vi "P1, P2, O2 Calculations.vi"(9 "O2 Voltage":dbl, 10 "P2 Voltage":dbl, 11 "P1 Voltage":dbl) -> (1 "O2":dbl, 2 "P2 Pressure":dbl, 3 "P1 Pressure":dbl)   [LabVIEW 2018]
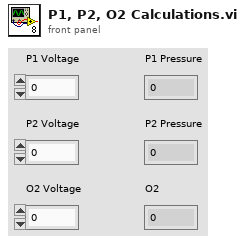
[diagram p1: front panel]
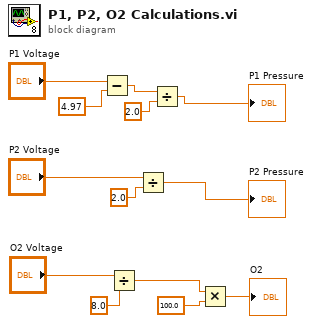
[diagram p0: block diagram]
diagram:
  n1 = Subtract(x="P1 Voltage", y=4.97 ("minimum value")) -> (x-y=w6:dbl)
  n2 = Divide(x="O2 Voltage", y=8.0 ("minimum value")) -> (x/y=w10:dbl)
  n3 = Divide(x="P2 Voltage", y=2.0 ("minimum value")) -> (x/y=→"P2 Pressure":dbl)
  n4 = Divide(x=w6, y=2.0 ("minimum value")) -> (x/y=→"P1 Pressure":dbl)
  n5 = Multiply(x=w10, y=100.0 ("minimum value")) -> (x*y=→"O2":dbl)
